vi "RSZVB Channel Add Trace Diagram Area.vi"(5 "Channel (1)":i32=1, 6 "Trace Name (Trc1)":string="Trc1", 7 "Channel Name (Ch1)":string="Ch1", 8 "error in (no error)":errorcluster {"code" format="%.0x"}, 9 "Window (Trace) (1)":i32=1, 10 "Window (1)":i32=1, 11 "VISA session":refnum<visa-resource-name>) -> (0 "error out":errorcluster {"code" format="%.0x"}, 3 "dup VISA session":refnum<visa-resource-name>)   [LabVIEW 2011]
doc: "This VI creates a new channel and a new trace, which is displayed in a new diagram area. The new channel settings (including a possible channel calibration) is preset to the default settings; the trace is created with the default trace settings.\n\nRemote-control command(s):\nCONFigure:CHANnel<Ch>[:STATe] ON\nCONFigure:CHANnel<Ch>:NAME '<string>'\nCALCulate<Ch>:PARameter:SDEFine '<string>', 'S21'\nDISPlay:WINDow<Wnd>:STATe ON\nDISPlay:WINDow<Wnd>:TRACe<WndTr>:FEED '<string>'"
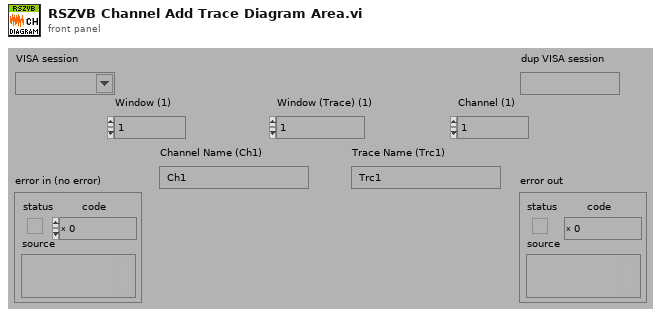
[diagram p1: front panel]
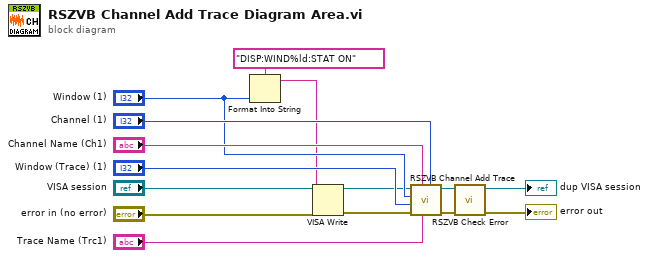
[diagram p0: block diagram]
diagram:
  n1 = Format Into String(format string="DISP:WIND%ld:STAT ON", "Window (1)") -> (resulting string=w1:string)  [unwired: 2 in, 1 out]
  n2 = VISA Write(VISA resource name="VISA session", write buffer=w1, error in (no error)="error in (no error)") -> (VISA resource name out=w5:refnum<visa-resource-name>, error out=w4:errorcluster)  [unwired: 1 out]
  n3 = call "RSZVB Channel Add Trace.vi"("Channel (1)"="Channel (1)", "Trace Name (Trc1)"="Trace Name (Trc1)", "Channel Name (Ch1)"="Channel Name (Ch1)", "error in (no error)"=w4, "Window (Trace) (1)"="Window (Trace) (1)", "Window (1)"="Window (1)", "VISA session"=w5) -> ("error out"=w7:errorcluster, "dup VISA session"=w6:refnum<visa-resource-name>)  [unwired: 3 in]
  n4 = call "RSZVB Check Error.vi"("error in (no error)"=w7, "VISA session"=w6) -> ("error out"=→"error out":errorcluster, "dup VISA session"=→"dup VISA session":refnum<visa-resource-name>)  [unwired: 8 in]
